vi "Read Per-Site Ref Mic LUT INI File.vi"(0 "LUT INI File Path":path, 5 "Site Number":i32, 11 "error in (no error)":errorcluster) -> (4 "Found?":bool, 6 "Serial Number":u32, 8 "Calibration File Name":string, 15 "error out":errorcluster)   [LabVIEW 2020]
uses:
  <vilib>/Utility/config.llb/Read Key (U32).vi
  <vilib>/Utility/config.llb/Read Key (String).vi
  <vilib>/Utility/config.llb/NI_LVConfig.lvlib
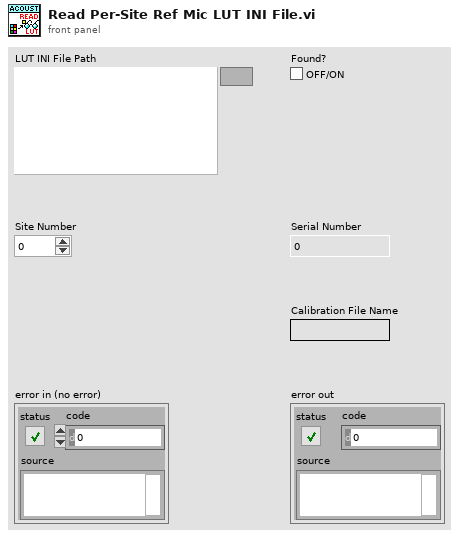
[diagram p1: front panel]
types:
  T1 = typedef "NI_LVConfig.lvlib/Config Data RefNum.ctl" = refnum<k1>
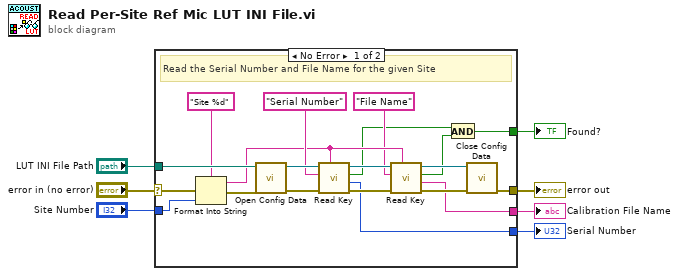
[diagram p0: block diagram]
diagram:
  n1 = case shown="No Error" "error in (no error)" {
    selector: "error in (no error)" -> [w24 w28]
    tunnel: [w14 w28] -> w7
    tunnel: "LUT INI File Path" -> [w27 _]
    tunnel: "Site Number" -> [w22 _]
    tunnel: [w12 _] -> w3
    tunnel: [w11 _] -> w2
    tunnel: [w8 _] -> w1
    frame No Error {
      # "Read the Serial Number and File Name for the given Site"
      n2 = Format Into String(format string="Site %d", error in=w24, w22) -> (resulting string=w17:string, error out=w23:errorcluster)  [unwired: 1 in]
      n3 = call <vilib>:"Open Config Data.vi"("error in (no error)"=w23, "configuration file path"=w27) -> ("error out"=w26:errorcluster, "refnum"=w25:T1)  [unwired: 7 in, 1 out]
      n4 = call-poly <vilib>:"Read Key.vi"("section"=w17, "error in (no error)"=w26, "key"="Serial Number" ("section"), "refnum"=w25) -> ("error out"=w19:errorcluster, "value"=w12:u32, "found?"=w10:bool, "refnum out"=w18:T1)  [unwired: 4 in]
      n5 = call-poly <vilib>:"Read Key.vi"("section"=w17, "error in (no error)"=w19, "key"="File Name" ("section"), "refnum"=w18) -> ("error out"=w15:errorcluster, "value"=w11:string, "found?"=w9:bool, "refnum out"=w13:T1)  [unwired: 4 in]
      n6 = And(x=w10, y=w9) -> (x .and. y?=w8:bool)
      n7 = call <vilib>:"Close Config Data.vi"("error in (no error)"=w15, "refnum"=w13) -> ("error out"=w14:errorcluster)  [unwired: 8 in, 1 out]
    }
    frame Error {
      # "Error case - Do Nothing"
    }
  }
  "error out" <- w7
  "Calibration File Name" <- w2
  "Serial Number" <- w3
  "Found?" <- w1
